vi "Actor Core.vi"(8 "error in":errorcluster, 11 "BuildServer in":refnum<class "BuildServer.lvclass">) -> (0 "error out":errorcluster, 3 "Actor out":refnum<class "Actor.lvclass">)   [LabVIEW 2017, in "BuildServer.lvlib" / "BuildServer.lvclass"]
doc: "(<B>Filename</B>: Actor Framework.lvlib:Actor.lvclass:Actor Core.vi)\n\nReceives messages to the actor, reacts to them, and initiates any error handling that may shut the actor down.\n\nDescendant classes may override this VI to append parallel tasks for the actor to complete while it handles messages. Overrides use the Call Parent Method node."
uses:
  BuildServer.lvclass
  C:/Users/Public/Documents/wc/BuildFarm/src/LabVIEW/vi.lib/BenjaminR/Build Farm/Actors/Framework/Actor wUI/Actor wUI.lvclass
  C:/Program Files (x86)/National Instruments/LabVIEW 2017/vi.lib/ActorFramework/Actor/Actor.lvclass
  C:/Users/Public/Documents/wc/BuildFarm/src/LabVIEW/vi.lib/BenjaminR/Build Farm/Actors/Framework/Actor wHelper/Actor wHelper.lvclass
  <vilib>/ActorFramework/Actor/Actor.lvclass
  ProjectOrganization.ctl
  Framework/Actor wUI/Actor wUI.lvclass/Actor wUI.ctl
  BuildServer.lvclass/BuildServer.ctl
  <vilib>/ActorFramework/Actor/Actor.lvclass/Actor.ctl
  <vilib>/ActorFramework/Message Enqueuer/Message Enqueuer.lvclass/Message Enqueuer.ctl
  Framework/Actor wHelper/Actor wHelper.lvclass/Actor wHelper.ctl
  <vilib>/Utility/sysdir.llb/System Directory Type.ctl
  BuildServer Messages/Add LVProject Msg/Add LVProject Msg.lvclass/Add LVProject Msg.ctl
  BuildServer Messages/Remove Tasks Msg/Remove Tasks Msg.lvclass/Remove Tasks Msg.ctl
  BuildServer Messages/Update Project Organization Msg/Update Project Organization Msg.lvclass/Update Project Organization Msg.ctl
  BuildServer Messages/Sort TaskView Msg/Sort TaskView Msg.lvclass/Sort TaskView Msg.ctl
  BuildServer Messages/Task Update Message Msg/Task Update Message Msg.lvclass/Task Update Message Msg.ctl
  BuildServer Messages/Launch Task Settings Msg/Launch Task Settings Msg.lvclass/Launch Task Settings Msg.ctl
  BuildServer Messages/Worker List Menu Selection Msg/Worker List Menu Selection Msg.lvclass/Worker List Menu Selection Msg.ctl
  Framework/Actor wHelper/Read StopHelperLoop Reg Ref.vi
  Framework/Actor wUI/Write UI Ref.vi
  <vilib>/ActorFramework/Message Enqueuer/Enqueue.vi
  <vilib>/ActorFramework/Message Enqueuer/Init from Existing Queue.vi
  BuildServer Messages/Send Tasks To Workers Msg/Send Tasks To Workers Msg.lvclass
  C:/Program Files (x86)/National Instruments/LabVIEW 2017/vi.lib/ActorFramework/Message/Message.lvclass
  BuildServer Messages/Start Tasks Msg/Start Tasks Msg.lvclass
  BuildServer Messages/Add LVProject Msg/Add LVProject Msg.lvclass
  BuildServer Messages/Remove Tasks Msg/Remove Tasks Msg.lvclass
  BuildServer Messages/Update Project Organization Msg/Update Project Organization Msg.lvclass
  BuildServer Messages/Sort TaskView Msg/Sort TaskView Msg.lvclass
  BuildServer Messages/Task Update Message Msg/Task Update Message Msg.lvclass
  BuildServer Messages/Stop Worker Msg/Stop Worker Msg.lvclass
  BuildServer Messages/Launch Task Settings Msg/Launch Task Settings Msg.lvclass
  BuildServer Messages/Worker List Menu Selection Msg/Worker List Menu Selection Msg.lvclass
  BuildServer Messages/Cancel Tasks Msg/Cancel Tasks Msg.lvclass
  <vilib>/ActorFramework/Message Priority Queue/Priority Enqueue.vi
  Get New Worker Event.vi
  Get Msg Update Event.vi
  <vilib>/ActorFramework/Message Enqueuer/Message Enqueuer.lvclass
  Framework/Actor wHelper/Actor wHelper.lvclass
  BuildServer Messages/Remove LVProject Msg/Remove LVProject Msg.lvclass
  BuildServer Messages/Add Tasks Msg/Add Tasks Msg.lvclass
panel:
  in  "tasksSend":bool
  in  "projectsDelete":bool
  in  "tasksAdd":bool
  in  "projectsOpen":bool
  in  "tasksRemove":bool
  in  "workerKill":bool
  in  "taskSettings":bool
  in  "taskCancel":bool
  in  "taskStart":bool
  in  "projectOrganization":T1
  in  "ProjectsView":string[](tree)
  in  "TasksView":i32[](listbox)
  out "#proc":i32 caption="# of logical processors"
  out "WorkerList":string[][](array[string])
  out "Status":string
  # "LabVIEW Projects"
  # "Tasks"
  # "Workers"
  # "Status"
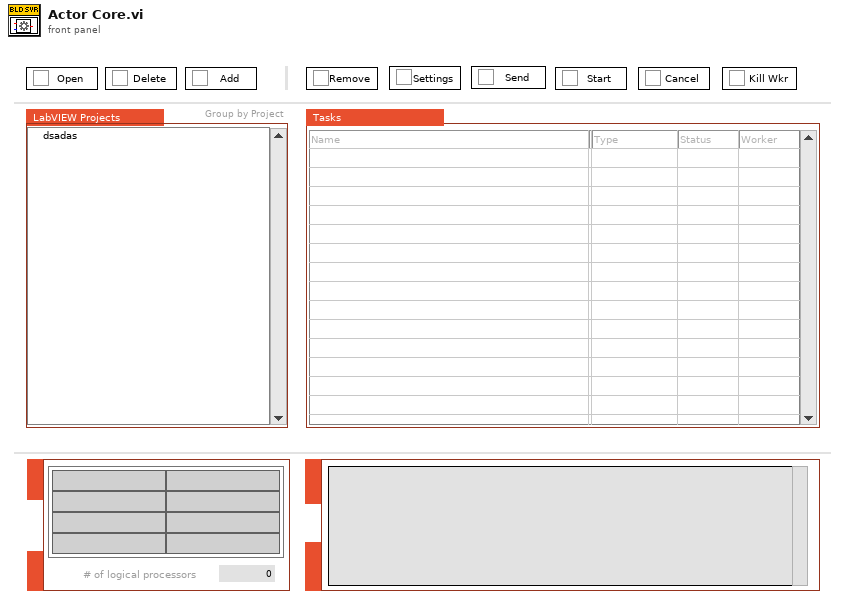
[diagram p1: front panel]
types:
  T1 = typedef "BuildServer.lvlib/BuildServer.lvclass/ProjectOrganization.ctl" = enum16{"Group by Project", "Group by Target", "Group by Type", "Group by Name"}
  T2 = cluster{"Properties:StopHelperLoop Reg Ref":refnum<event-registration>, "Properties:Msg Update Event":refnum<event-registration>, "Properties:New Worker Event":refnum<event-registration>}
  T3 = typedef "System Directory Type.ctl" = i32
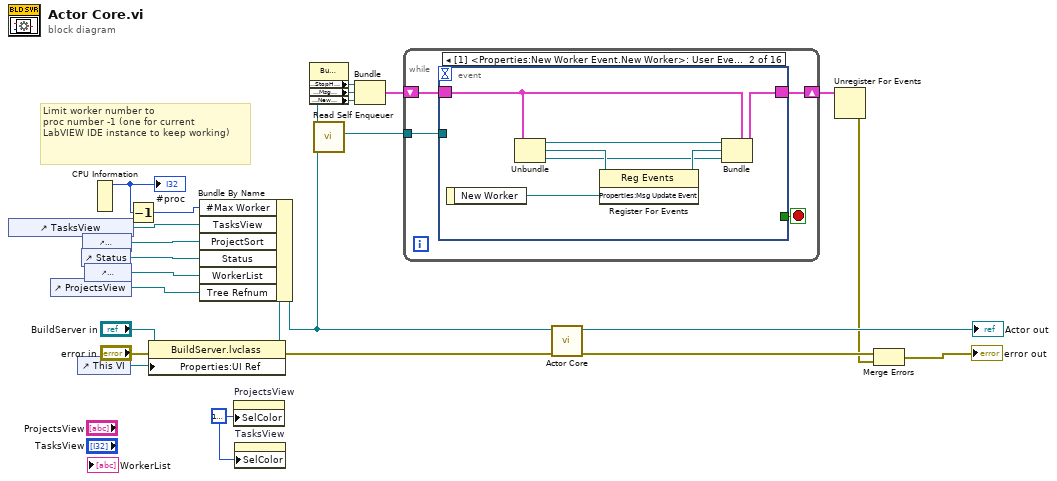
[diagram p0: block diagram]
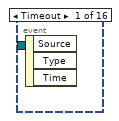
[diagram p2: hidden frame]
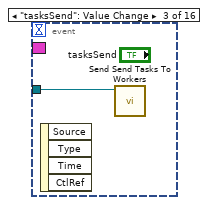
[diagram p3: hidden frame]
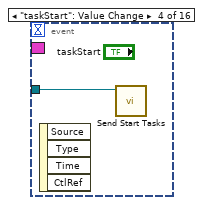
[diagram p4: hidden frame]
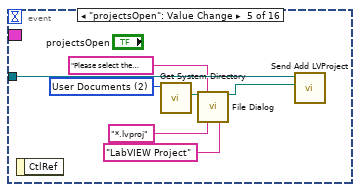
[diagram p5: hidden frame]
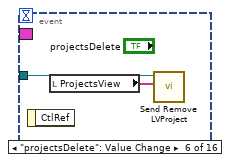
[diagram p6: hidden frame]
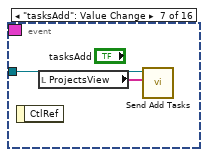
[diagram p7: hidden frame]
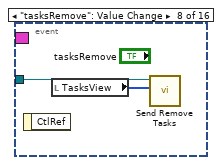
[diagram p8: hidden frame]
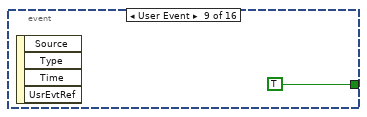
[diagram p9: hidden frame]
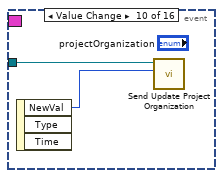
[diagram p10: hidden frame]
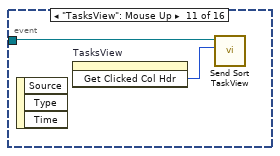
[diagram p11: hidden frame]
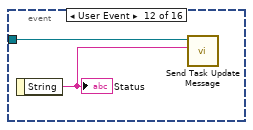
[diagram p12: hidden frame]
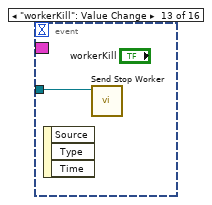
[diagram p13: hidden frame]
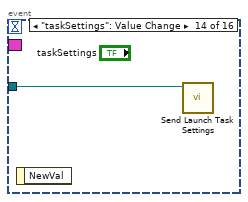
[diagram p14: hidden frame]
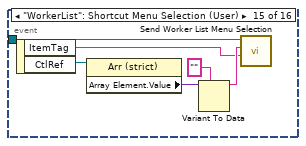
[diagram p15: hidden frame]
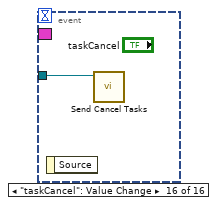
[diagram p16: hidden frame]
diagram:
  w13 = u32 16777224 ("Selection Color")
  # "Limit worker number to\nproc number -1 (one for current\nLabVIEW IDE instance to keep working)"
  n1 = control-ref of="TasksView"() -> (w14:refnum<vi>)
  n2 = control-ref of="ProjectsView"() -> (w19:refnum<vi>)
  n3 = control-ref of="This VI"() -> (w3:refnum<vi>)
  n4 = control-ref of="Status"() -> (w16:refnum<vi>)
  n5 = control-ref of="projectOrganization"() -> (w15:refnum<vi>)
  n6 = control-ref of="WorkerList"() -> (w17:refnum<vi>)
  n7 = CPU Information() -> (4:w10:i32)  [unwired: 3 out]
  "#proc" <- w10
  n8 = Decrement(x=w10) -> (x-1=w9:i32)
  n9 = property class="BuildServer.lvclass"(reference="BuildServer in", error in="error in", "Properties:UI Ref"=w3) -> (reference out=w5:refnum<class "BuildServer.lvclass">, error out=w1:errorcluster)
  n10 = Bundle By Name(cluster=w5, "#Max Worker"=w9, "TasksView"=w14, "ProjectSort"=w15, "Status"=w16, "WorkerList"=w17, "Tree Refnum"=w19) -> (w2:refnum<class "BuildServer.lvclass">)
  n11 = property on="ProjectsView" class="Tree (strict)"("SelColor"=w13) -> ()  [unwired: 2 in, 2 out]
  n12 = property on="TasksView" class="MCListbox (strict)"("SelColor"=w13) -> ()  [unwired: 2 in, 2 out]
  n13 = property class="BuildServer.lvclass"(reference=w2) -> ("Properties:StopHelperLoop Reg Ref"=w21:refnum<event-registration>, "Properties:Msg Update Event"=w8:refnum<event-registration>, "Properties:New Worker Event"=w6:refnum<event-registration>)  [unwired: 1 in, 2 out]
  n14 = call <vilib>:"Read Self Enqueuer.vi"("Actor"=w2) -> ("Self Enqueuer"=w18:refnum<class "Message Enqueuer.lvclass">)  [unwired: 10 in]
  n15 = Bundle("Properties:StopHelperLoop Reg Ref"=w21, "Properties:Msg Update Event"=w8, "Properties:New Worker Event"=w6) -> (w20:T2)  [unwired: 1 in]
  n16 = while {
    tunnel: w18 -> [w26]
    shift-right: [w25] -> w7
    shift-left: w20 -> [w27]
    stop <- w28 stop-if-true
    n17 = event shown="[1] <Properties:New Worker Event.New Worker>: User Event" {
      selector: w27 -> [_ w35 _ _ _ _ _ _ _ _ _ _ _ _ _ _]
      dyn-events: [_ w33 _ _ _ _ _ _ _ _ _ _ _ _ _ _] -> w25
      timeout: _ -> [_ _ _ _ _ _ _ _ _ _ _ _ _ _ _ _]
      tunnel: [_ _ _ _ _ _ _ _ TRUE ("Discard?") _ _ _ _ _ _ _] -> w28
      tunnel: w26 -> [_ _ w36 w37 w44 w46 w48 w50 _ w53 w55 w57 w58 w59 w62 w66]
      event Timeout {
        n18 = event-data() -> ()  [unwired: 1 in, 3 out]
      }
      event User Event {
        n19 = event-data() -> ("New Worker"=w29:refnum<user-event>)  [unwired: 1 in]
        n20 = Unbundle(w35) -> ("Properties:StopHelperLoop Reg Ref"=w32:refnum<event-registration>, "Properties:Msg Update Event"=w34:refnum<event-registration>, "Properties:New Worker Event"=w30:refnum<event-registration>)
        n21 = register-events(reference=w34, w29) -> (reference out=w31:refnum<event-registration>)  [unwired: 1 in, 1 out]
        n22 = Bundle(cluster=w35, "Properties:StopHelperLoop Reg Ref"=w32, "Properties:Msg Update Event"=w31, "Properties:New Worker Event"=w30) -> (w33:T2)
      }
      event "tasksSend": Value Change {
        n23 = event-data() -> ()  [unwired: 1 in, 4 out]
        n24 = call "Send Send Tasks To Workers.vi"("Message Enqueuer in"=w36) -> ()  [unwired: 9 in, 2 out]
      }
      event "taskStart": Value Change {
        n25 = event-data() -> ()  [unwired: 1 in, 4 out]
        n26 = call "Send Start Tasks.vi"("Message Enqueuer in"=w37) -> ()  [unwired: 9 in, 2 out]
      }
      event "projectsOpen": Value Change {
        w42 = T3 2 items=["User Home"=0, "User Desktop"=1, "User Documents"=2, "User Application Data"=3, "User Preferences"=4, "User Temporary"=5, "Public Documents"=6, "Public Application Data"=7, "Public Preferences"=8, "Public Cache"=13, "System Core Libraries"=9, "System Installed Libraries"=10, "Application Files"=11, "Boot Volume Root"=12] ("system directory type")
        n27 = event-data() -> ()  [unwired: 1 in, 1 out]
        n28 = call <vilib>:"Get System Directory.vi"("system directory type"=w42) -> ("system directory"=w43:path)  [unwired: 10 in]
        n29 = call "File Dialog"("start path"=w43, "prompt"="Please select the LabVIEW project you want to load.", "pattern (all files)"="*.lvproj", "pattern label"="LabVIEW Project") -> ("selected path"=w38:path)  [unwired: 8 in, 3 out]
        n30 = call "Send Add LVProject.vi"("Project Path"=w38, "Message Enqueuer in"=w44) -> ()  [unwired: 8 in, 2 out]
      }
      event "projectsDelete": Value Change {
        n31 = event-data() -> ()  [unwired: 1 in, 1 out]
        n32 = local read "ProjectsView"() -> (w45:string[])
        n33 = call "Send Remove LVProject.vi"("User Selections"=w45, "Message Enqueuer in"=w46) -> ()  [unwired: 8 in, 2 out]
      }
      event "tasksAdd": Value Change {
        n34 = event-data() -> ()  [unwired: 1 in, 1 out]
        n35 = local read "ProjectsView"() -> (w47:string[])
        n36 = call "Send Add Tasks.vi"("User Selections"=w47, "Message Enqueuer in"=w48) -> ()  [unwired: 8 in, 2 out]
      }
      event "tasksRemove": Value Change {
        n37 = event-data() -> ()  [unwired: 1 in, 1 out]
        n38 = local read "TasksView"() -> (w49:i32[])
        n39 = call "Send Remove Tasks.vi"("User Selections"=w49, "Message Enqueuer in"=w50) -> ()  [unwired: 8 in, 2 out]
      }
      event User Event {
        n40 = event-data() -> ()  [unwired: 1 in, 4 out]
      }
      event Value Change {
        n41 = event-data() -> ("NewVal"=w52:T1)  [unwired: 1 in, 2 out]
        n42 = call "Send Update Project Organization.vi"("ProjectOrganization"=w52, "Message Enqueuer in"=w53) -> ()  [unwired: 8 in, 2 out]
      }
      event "TasksView": Mouse Up {
        n43 = event-data() -> ()  [unwired: 1 in, 3 out]
        n44 = invoke on="TasksView" class="MCListbox (strict)" method="Get Clicked Col Hdr"() -> ("Get Clicked Column Header"=w54:i32)  [unwired: 3 in, 2 out]
        n45 = call "Send Sort TaskView.vi"("Clicked Column"=w54, "Message Enqueuer in"=w55) -> ()  [unwired: 8 in, 2 out]
      }
      event User Event {
        n46 = event-data() -> ("String"=w56:string)  [unwired: 1 in]
        "Status" <- w56
        n47 = call "Send Task Update Message.vi"("Task Update Message"=w56, "Message Enqueuer in"=w57) -> ()  [unwired: 8 in, 2 out]
      }
      event "workerKill": Value Change {
        n48 = event-data() -> ()  [unwired: 1 in, 3 out]
        n49 = call "Send Stop Worker.vi"("Message Enqueuer in"=w58) -> ()  [unwired: 9 in, 2 out]
      }
      event "taskSettings": Value Change {
        n50 = event-data() -> ()  [unwired: 1 in, 1 out]
        n51 = call "Send Launch Task Settings.vi"("Message Enqueuer in"=w59) -> ()  [unwired: 9 in, 2 out]
      }
      event "WorkerList": Shortcut Menu Selection (User) {
        n52 = event-data() -> ("ItemTag"=w60:string, "CtlRef"=w65:refnum<vi>)  [unwired: 1 in]
        n53 = property class="Arr (strict)"(reference=w65) -> ("Array Element.Value"=w64:variant)  [unwired: 1 in, 2 out]
        n54 = Variant To Data(type="", Variant=w64) -> (data=w61:string)  [unwired: 1 in, 1 out]
        n55 = call "Send Worker List Menu Selection.vi"("Menu Item Tag"=w60, "Worker Name"=w61, "Message Enqueuer in"=w62) -> ()  [unwired: 7 in, 2 out]
      }
      event "taskCancel": Value Change {
        n56 = event-data() -> ()  [unwired: 1 in, 1 out]
        n57 = call "Send Cancel Tasks.vi"("Message Enqueuer in"=w66) -> ()  [unwired: 9 in, 2 out]
      }
    }
  }
  n58 = call-parent "Actor Core.vi"("error in"=w1, "Actor in"=w2) -> ("error out"=w24:errorcluster, "Actor out"=→"Actor out":refnum<class "Actor.lvclass">)  [unwired: 8 in]
  n59 = Unregister For Events(event registration refnum=w7) -> (error out=w11:errorcluster)  [unwired: 1 in]
  n60 = Merge Errors(w24, w11) -> (→"error out":errorcluster)
